vi "Select Bests (SubVI).vi"(6 "error out 3":errorcluster, 7 "Candidate beads":dbl[][](array[numeric]), 8 "CorrelationTreshold":dbl=0.6, 9 "Roi size":i32=2, 10 "Proximity (ROI size units)":dbl=0.45) -> (2 "Good Beads":dbl[][](array[numeric]), 4 "error out 2":errorcluster)   [LabVIEW 2011, in "OfflineTracker.lvlib"]
doc: "This vi takes the first n elements still close enough to the first value. It assumes a pre-sorted array, max first. JacobKers09"
uses:
  OfflineTracker.lvlib
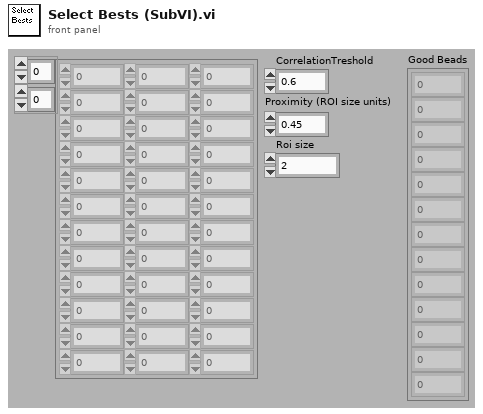
[diagram p1: front panel]
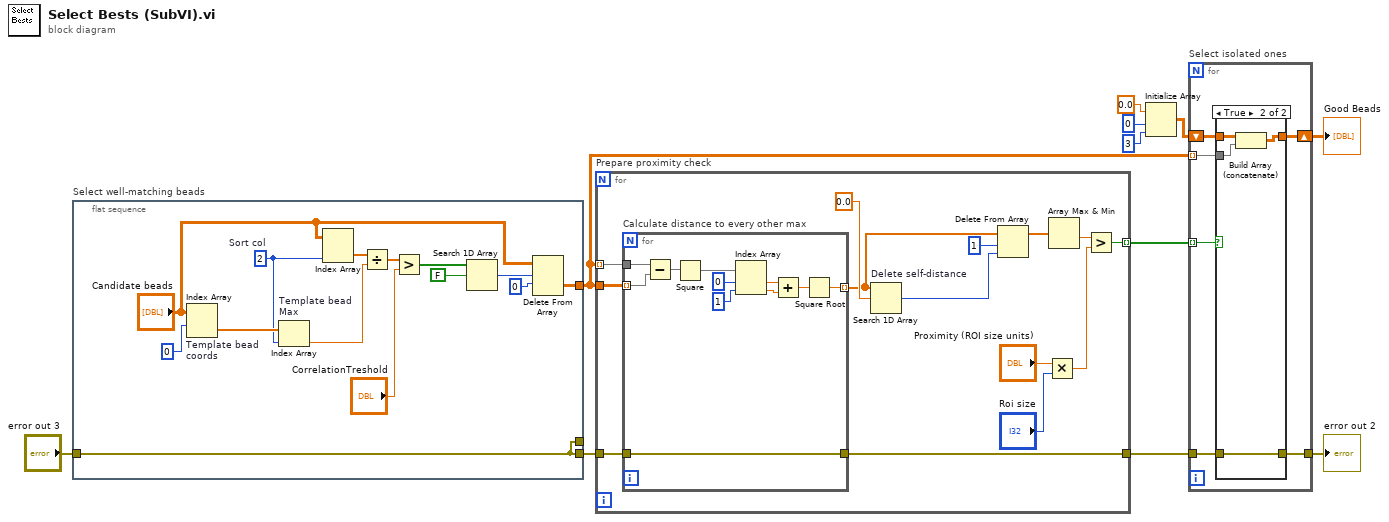
[diagram p0: block diagram]
diagram:
  n1 = flat-sequence "Select well-matching beads" {
    tunnel: [w24] -> w11
    tunnel: [w12] -> _
    tunnel: "error out 3" -> [w12]
    tunnel: [w12] -> w1
    frame #0 {
      w14 = 2  # Sort col
      n2 = Index Array "Template bead \ncoords"(array="Candidate beads", index (row)=0) -> (element=w22:dbl[])  [unwired: 1 in]
      n3 = Index Array "Template bead \nMax"(array=w22, index=w14) -> (element=w19:dbl)
      n4 = Index Array(array="Candidate beads", index (col)=w14) -> (element=w20:dbl[])  [unwired: 1 in]
      n5 = Divide(x=w20, y=w19) -> (x/y=w21:dbl[])
      n6 = Greater?(x=w21, y="CorrelationTreshold") -> (0:w13:bool[])
      n7 = Search 1D Array(1D array=w13, element=FALSE) -> (index of element=w17:i32)  [unwired: 1 out]
      n8 = Delete From Array(array="Candidate beads", length=w17, index (row)=0) -> (deleted portion=w24:dbl[][])  [unwired: 1 in, 1 out]
    }
  }
  n9 = for "Prepare proximity check" {
    tunnel: w11 -> [w38] mode=indexing
    tunnel: w11 -> [w39]
    tunnel: [w37] -> w8 mode=indexing
    tunnel: w1 -> [w27]
    tunnel: [w26] -> w3
    n10 = for "Calculate distance to every other max" {
      tunnel: w39 -> [w49] mode=indexing
      tunnel: w38 -> [w50]
      tunnel: [w41] -> w33 mode=indexing
      tunnel: w27 -> [w40]
      tunnel: [w40] -> w26
      n11 = Subtract(x=w50, y=w49) -> (x-y=w48:dbl[])
      n12 = Square(x=w48) -> (x^2=w47:dbl[])
      n13 = Index Array(array=w47, index #1=0 ("length"), index #2=1 ("index")) -> (element #1=w44:dbl, element #2=w43:dbl)
      n14 = Add(x=w44, y=w43) -> (x+y=w42:dbl)
      n15 = Square Root(x=w42) -> (sqrt(x)=w41:dbl)
    }
    n16 = Search 1D Array "Delete self-distance"(1D array=w33, element=0.0) -> (index of element=w35:i32)  [unwired: 1 out]
    n17 = Delete From Array(array=w33, length=1, index=w35) -> (array with subset deleted=w32:dbl[])  [unwired: 1 out]
    n18 = Multiply(x="Proximity (ROI size units)", y="Roi size") -> (x*y=w30:dbl)
    n19 = Array Max & Min(array=w32) -> (min value=w31:dbl)  [unwired: 3 out]
    n20 = Greater?(x=w31, y=w30) -> (0:w37:bool)
  }
  n21 = Initialize Array(0.0 ("element"), 0 ("dimension size"), 3 ("dimension size")) -> (w7:dbl[][])
  n22 = for "Select isolated ones" {
    tunnel: w11 -> [w55] mode=indexing
    tunnel: w8 -> [w53] mode=indexing
    shift-right: [w54] -> w9
    shift-left: w7 -> [w56]
    tunnel: w3 -> [w52]
    tunnel: [w51] -> w10
    n23 = case shown="True" w53 {
      tunnel: w56 -> [w58 w62]
      tunnel: w55 -> [_ w61]
      tunnel: [w58 w60] -> w54
      tunnel: [w57 w59] -> w51
      tunnel: w52 -> [w57 w59]
      frame False {
      }
      frame True {
        n24 = Build Array (concatenate)(w62, w61) -> (w60:dbl[][])
      }
    }
  }
  "error out 2" <- w10
  "Good Beads" <- w9
